vi "MSEncoder SubVI SignalRemarksInit.vi"(11 "MSEncoder in":refnum<class "MSEncoder.lvclass">) -> (3 "MSEncoder out":refnum<class "MSEncoder.lvclass">)   [LabVIEW 2018, in "MSEncoder.lvclass"]
uses:
  MSEncoder.lvclass
  PublicSubVI/Class/SigInfo/SigInfo.ctl
  MSEncoder.lvclass/MSEncoder.ctl
  PublicSubVI/Class/SigInfo/SigInfo.lvclass
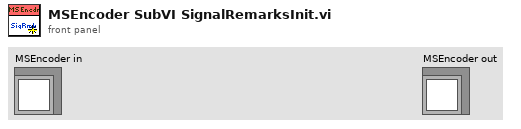
[diagram p1: front panel]
types:
  T1 = typedef "SigInfo.ctl" = enum16{"New mzList", "Set SigInfo", "Get SigInfo", "Append", "End"}
  T2 = cluster{"mzID":u64, "SignalInfo":cluster{"Label":string, "dt":dbl, "Length":u32, "RefVolt":dbl, "mzTable":cluster{"t":dbl[], "mz":dbl[], "beta":dbl[]}}[]}
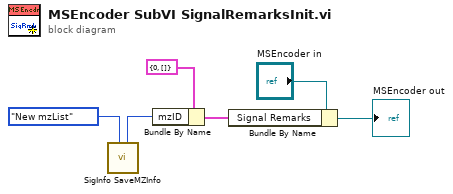
[diagram p0: block diagram]
diagram:
  n1 = call "SigInfo SaveMZInfo.vi"("Function"=SigInfo."New mzList") -> ("ID"=w2:u64)  [unwired: 8 in, 2 out]
  n2 = Bundle By Name(cluster=T2 {"mzID"=0, "SignalInfo"=[]} ("Signal Remarks"), "mzID"=w2) -> (w3:T2)
  n3 = Bundle By Name(cluster="MSEncoder in", "Signal Remarks"=w3) -> (→"MSEncoder out":refnum<class "MSEncoder.lvclass">)
